vi "FunctionToJson.vi"(8 "error in (no error)":errorcluster, 10 "Relative Bounds":cluster{"x":i32, "y":i32, "w":i32, "h":i32}, 11 "Function Ref In":refnum<vi>) -> (0 "error out":errorcluster, 3 "JSON":string)   [LabVIEW 2017]
doc: "Convert Function nodes to JSON"
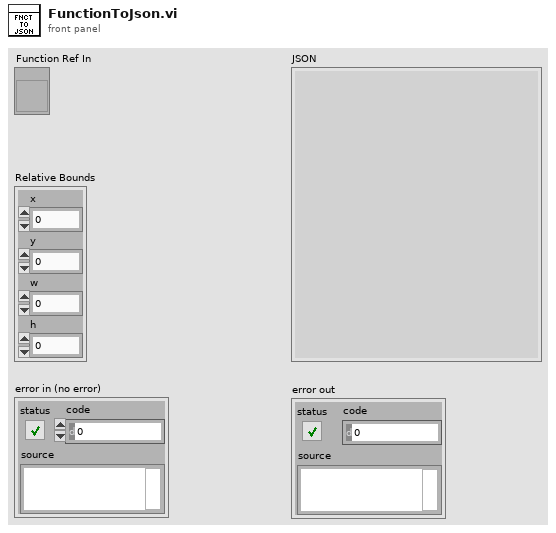
[diagram p1: front panel]
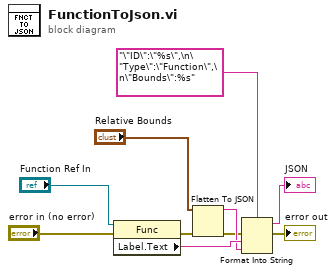
[diagram p0: block diagram]
diagram:
  n1 = property class="Func"(reference="Function Ref In", error in="error in (no error)") -> (error out=w3:errorcluster, "Label.Text"=w8:string)  [unwired: 1 out]
  n2 = Flatten To JSON(anything="Relative Bounds", error in (no error)=w3) -> (JSON string=w7:string, 11:w2:errorcluster)  [unwired: 1 in]
  n3 = Format Into String(format string="\"ID\":\"%s\",\n\"Type\":\"Function\",\n\"Bounds\":%s", error in=w2, w8, w7) -> (resulting string=→"JSON":string, error out=→"error out":errorcluster)  [unwired: 1 in]
